vi "RPi HMI Com.vi"(0 "Pump Data":T4={"Voltages"=[0.0, 0.05908203125, 0.06982421875, 0.05908203125, 0.06982421875, 0.0859375], "PumpCurrent"=[0.0015967955457961394, 0.0015950073791676203, 0.0015981739242389562, 0.0015920643549248493, 0.001590499709124895, 0.0015808510600251774], "Speed"=[0.0, 0.0, 0.0, 0.0, 0.0, 0.0], "ControllerCurrent"=[0.0, 0.0, 0.0, 0.0, 0.0, 0.0], "Pressure"=[0.0, 0.0, 0.0, 0.0, 0.0, 0.0], "Flow"=[0.0, 0.0, 0.0, 0.0, 0.0, 0.0], "Elapsed Time:"=[4074.9003000000002, 4074.9003000000002, 4074.9003000000002, 4074.9003000000002, 4074.9003000000002, 4074.9003000000002]} {"Elapsed Time:" format="%<%H:%M:%S>t"; "Speed" format="%#_4f"; "ControllerCurrent" format="%#.1g"; "Pressure" format="%#.0f"; "Flow" format="%#.0f"; "PumpCurrent" format="%#.1g"; "Voltages" format="%#.0f"}, 1 "Tank Data":T10 {"PS Actual (V):" format="%.2f"; "Temp1" format="%#_2g"; "Temp2" format="%#_2g"}, 2 "Power Relays":T9, 3 "Pump CMDs":dbl[](array[numeric]), 4 "HMI Header":T5, 5 "Tank CMDs":T6, 7 "HMI Tog Buttons":T7, 8 "RPi HMI Mode":T11, 9 "In Test":bool, 11 "Controller Config":T1) -> (14 "HMI Cluster":T3 {"Pump Data"."Elapsed Time:" format="%<%H:%M:%S>t"; "Pump Data"."Speed" format="%#_4f"; "Pump Data"."ControllerCurrent" format="%#.1g"; "Pump Data"."Pressure" format="%#.0f"; "Pump Data"."Flow" format="%#.0f"; "Pump Data"."PumpCurrent" format="%#.1g"; "Pump Data"."Voltages" format="%#.0f"})   [LabVIEW 2013]
uses:
  Controls/RPi HMI Mode.ctl
  Controls/Pump Data.ctl
  Controls/HMI Header.ctl
  Controls/Tank CMDs.ctl
  Controls/HMI Tog Buttons.ctl
  Controls/HMI Cluster.ctl
  Controls/HMI Mom Buttons.ctl
  Controls/Controller Config.ctl
  Type Defs/Controller Names.ctl
  <vilib>/Instr/_visa.llb/VISA Configure Serial Port (Instr).vi
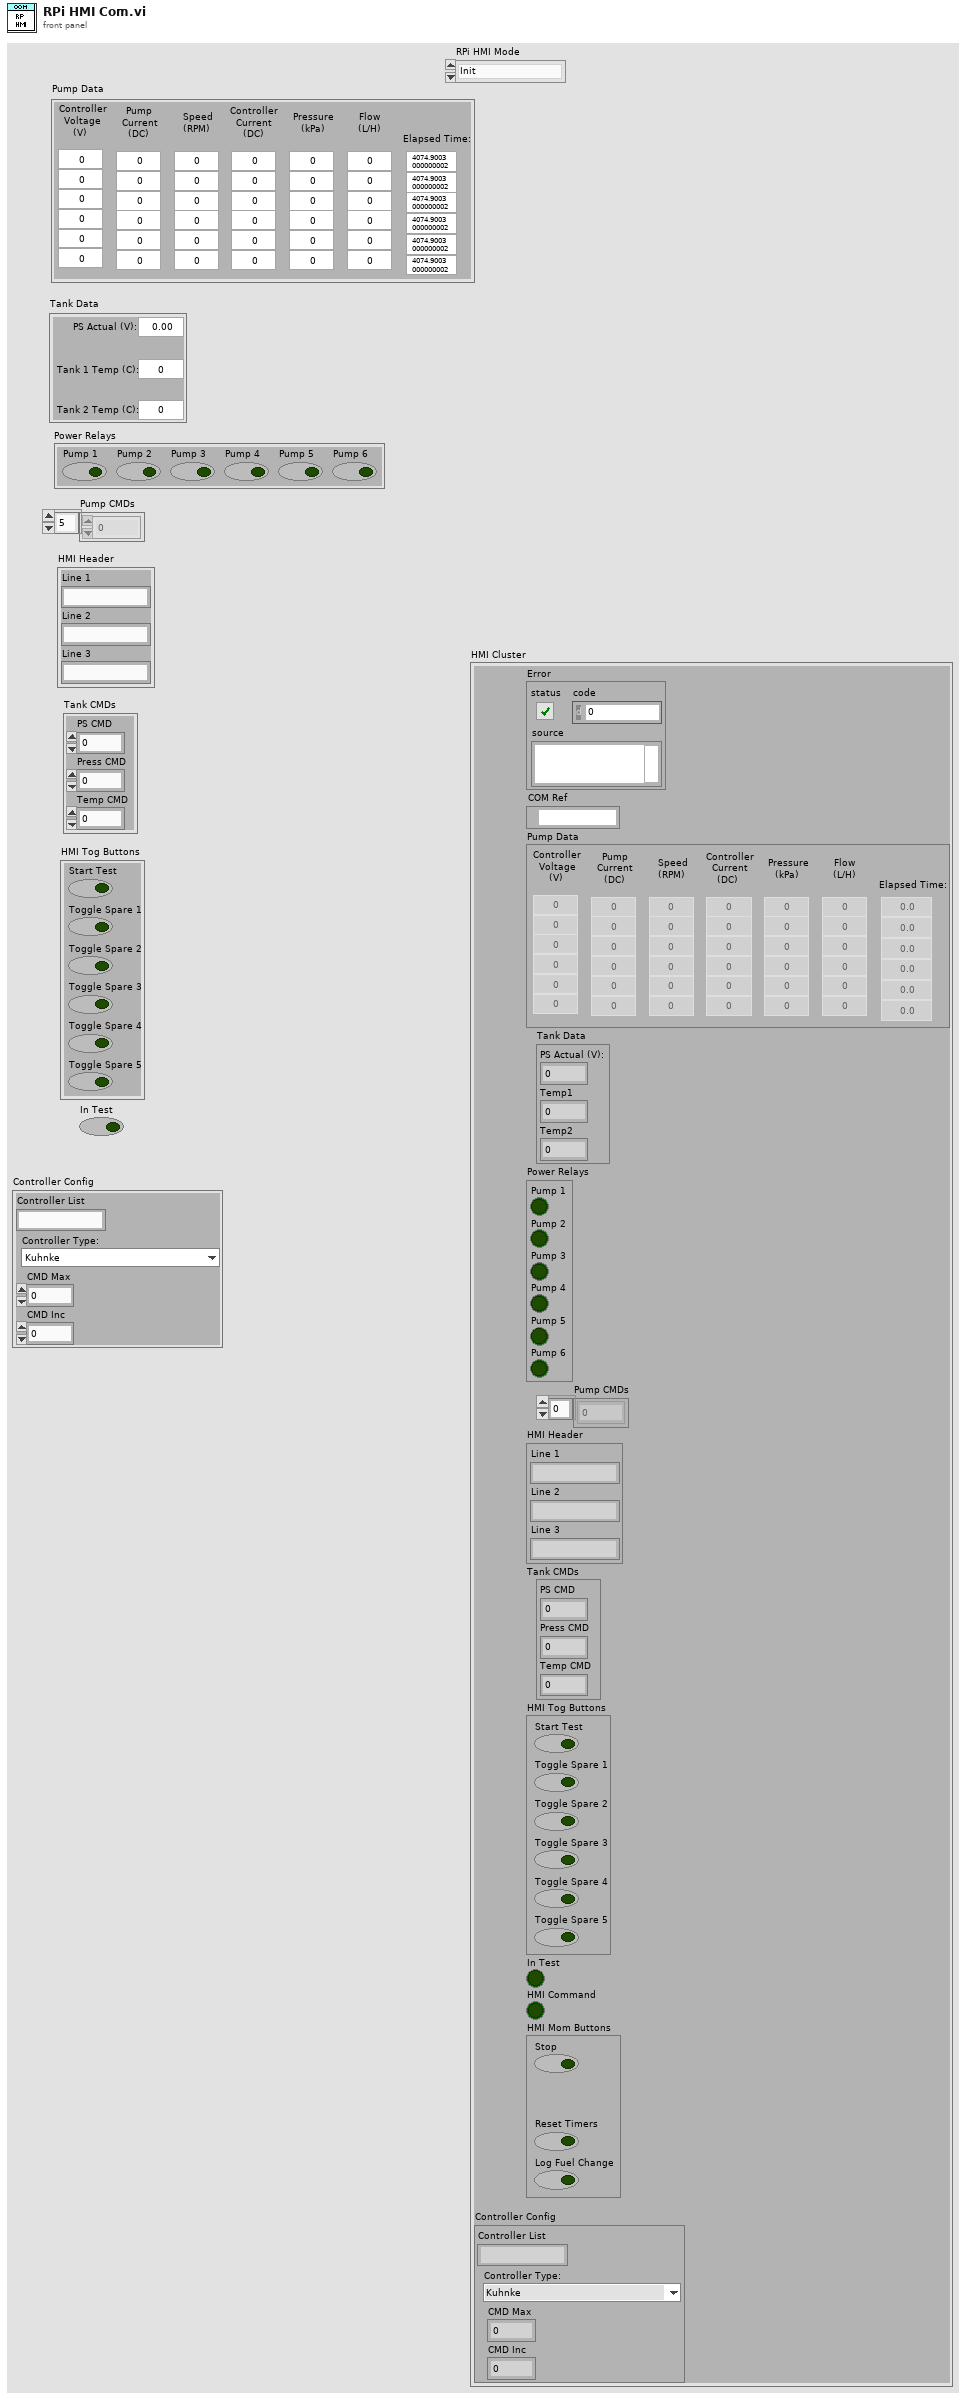
[diagram p1: front panel]
types:
  T1 = typedef "Controller Config.ctl" = cluster{"Controller List":string, "Controller Type:":T2, "CMD Max":i32, "CMD Inc":i32}
  T2 = typedef "Controller Names.ctl" = enum16{"Kuhnke", "Conti", "Hella CAN", "Helbako", "TI PWM", "PSA", "Hella DC Gas", "Hella DC Diesel", "8 Comm", "10 Comm", "8 Comm Hella", "10 Comm Hella", "8 Comm Omron", "10 Comm Omron", "8 Comm Nissan", "10 Comm Nissan"}
  T3 = typedef "HMI Cluster.ctl" = cluster{"Error":errorcluster, "COM Ref":refnum<visa-resource-name>, "Pump Data":T4, "Tank Data":cluster{"PS Actual (V):":dbl, "Temp1":dbl, "Temp2":dbl}, "Power Relays":cluster{"Pump 1":bool, "Pump 2":bool, "Pump 3":bool, "Pump 4":bool, "Pump 5":bool, "Pump 6":bool}, "Pump CMDs":dbl[], "HMI Header":T5, "Tank CMDs":T6, "HMI Tog Buttons":T7, "In Test":bool, "HMI Command":bool, "HMI Mom Buttons":T8, "Controller Config":T1}
  T4 = typedef "Pump Data.ctl" = cluster{"Voltages":dbl[], "PumpCurrent":dbl[], "Speed":dbl[], "ControllerCurrent":dbl[], "Pressure":dbl[], "Flow":dbl[], "Elapsed Time:":dbl[]}
  T5 = typedef "HMI Header.ctl" = cluster{"Line 1":string, "Line 2":string, "Line 3":string}
  T6 = typedef "Tank CMDs.ctl" = cluster{"PS CMD":dbl, "Press CMD":dbl, "Temp CMD":dbl}
  T7 = typedef "HMI Tog Buttons.ctl" = cluster{"Start Test":bool, "Toggle Spare 1":bool, "Toggle Spare 2":bool, "Toggle Spare 3":bool, "Toggle Spare 4":bool, "Toggle Spare 5":bool}
  T8 = typedef "HMI Mom Buttons.ctl" = cluster{"Stop":bool, "Reset Timers":bool, "Log Fuel Change":bool}
  T9 = cluster{"Pump 1":bool, "Pump 2":bool, "Pump 3":bool, "Pump 4":bool, "Pump 5":bool, "Pump 6":bool}
  T10 = cluster{"PS Actual (V):":dbl, "Temp1":dbl, "Temp2":dbl}
  T11 = typedef "RPi HMI Mode.ctl" = enum16{"Init", "Write Data", "Read from RPi", "Write to RPi"}
  T12 = cluster{"Tank CMDs[0]":dbl, "Tank CMDs[1]":dbl, "Tank CMDs[2]":dbl}
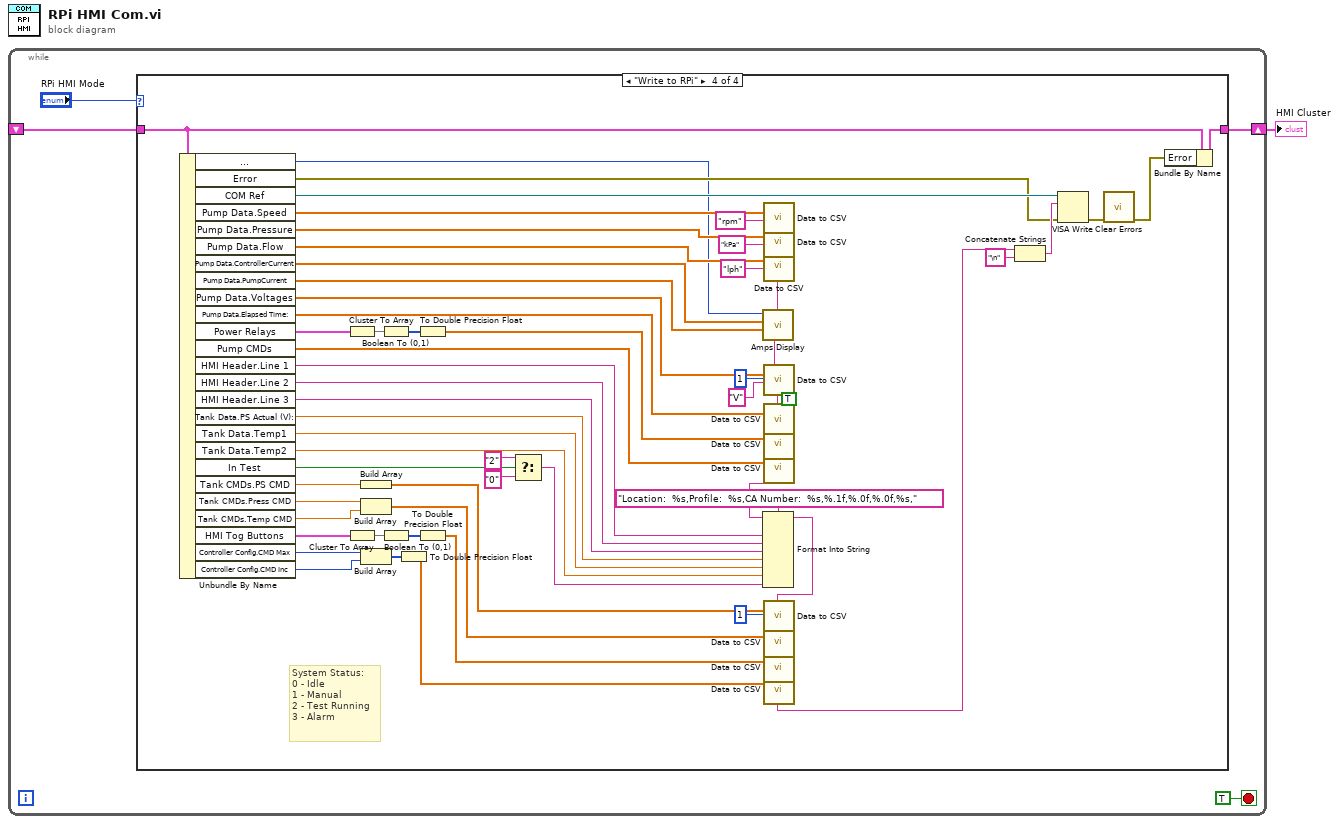
[diagram p0: block diagram]
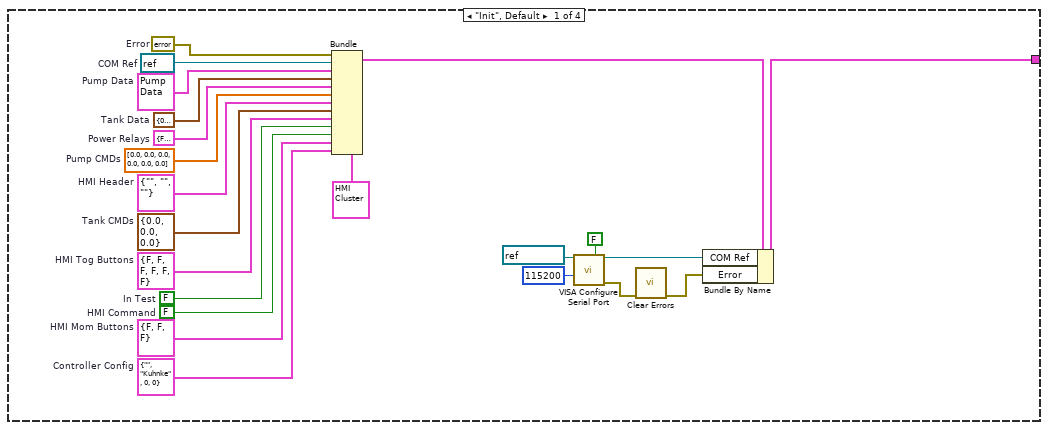
[diagram p2: hidden frame]
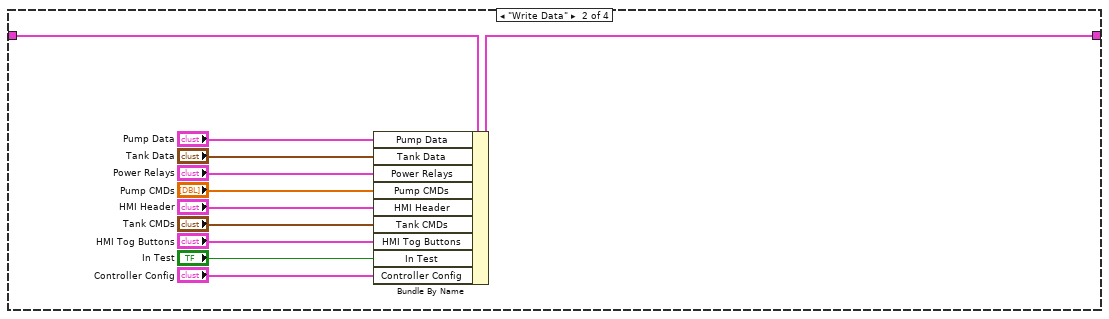
[diagram p3: hidden frame]
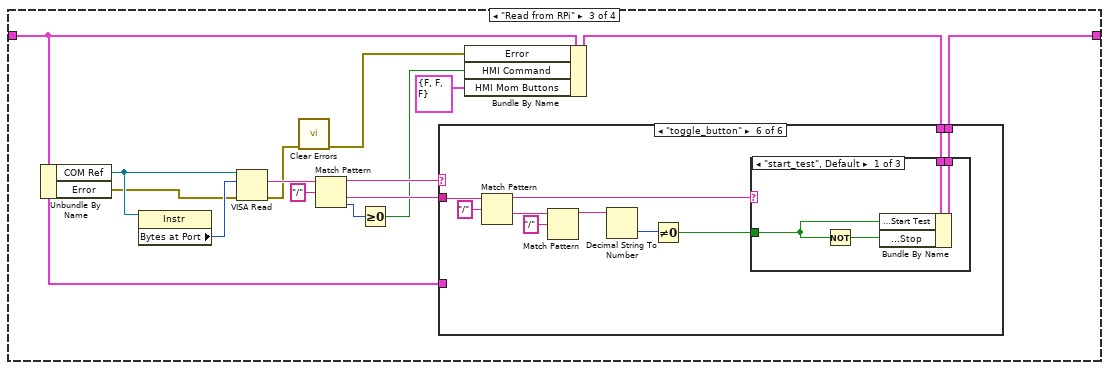
[diagram p4: hidden frame]
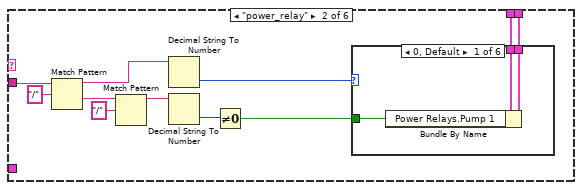
[diagram p6: hidden frame]
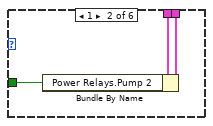
[diagram p7: hidden frame]
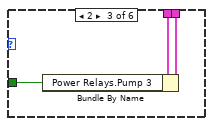
[diagram p8: hidden frame]
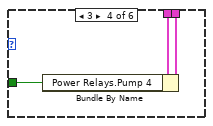
[diagram p9: hidden frame]
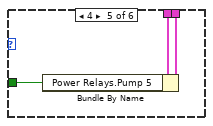
[diagram p10: hidden frame]
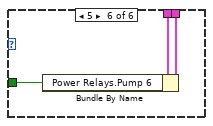
[diagram p11: hidden frame]
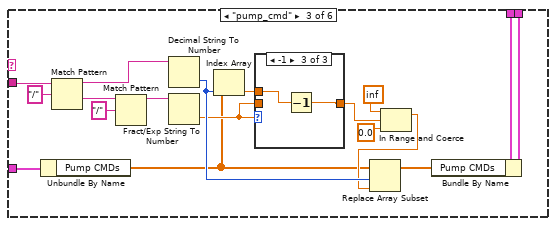
[diagram p12: hidden frame]
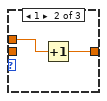
[diagram p14: hidden frame]
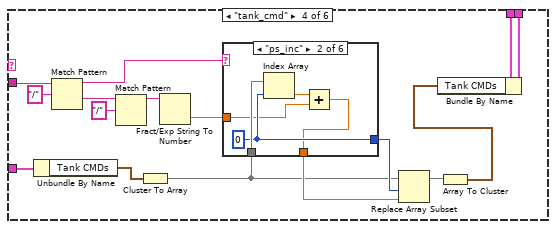
[diagram p15: hidden frame]
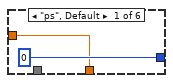
[diagram p16: hidden frame]
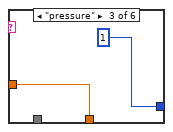
[diagram p17: hidden frame]
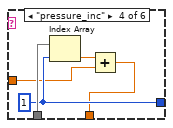
[diagram p18: hidden frame]
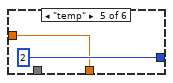
[diagram p19: hidden frame]
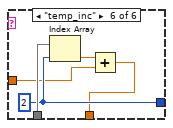
[diagram p20: hidden frame]
diagram:
  n1 = while {
    shift-right: [w3] -> w1
    shift-left: _ -> [w2]
    stop <- TRUE stop-if-true
    n2 = case shown="\"Write to RPi\"" "RPi HMI Mode" {
      tunnel: [w21 w37 w45 w189] -> w3
      tunnel: w2 -> [_ w38 w43 w190]
      frame "Init", Default {
        w6 = T1 {"Controller List"="", "Controller Type:"=enum."Kuhnke", "CMD Max"=0, "CMD Inc"=0}  # Controller Config
        w10 = T8 {"Stop"=FALSE, "Reset Timers"=FALSE, "Log Fuel Change"=FALSE}  # HMI Mom Buttons
        w11 = T9 {"Pump 1"=FALSE, "Pump 2"=FALSE, "Pump 3"=FALSE, "Pump 4"=FALSE, "Pump 5"=FALSE, "Pump 6"=FALSE}  # Power Relays
        w12 = FALSE  # HMI Command
        w13 = FALSE  # In Test
        w14 = T7 {"Start Test"=FALSE, "Toggle Spare 1"=FALSE, "Toggle Spare 2"=FALSE, "Toggle Spare 3"=FALSE, "Toggle Spare 4"=FALSE, "Toggle Spare 5"=FALSE}  # HMI Tog Buttons
        w15 = T6 {"PS CMD"=0.0, "Press CMD"=0.0, "Temp CMD"=0.0}  # Tank CMDs
        w16 = T5 {"Line 1"="", "Line 2"="", "Line 3"=""}  # HMI Header
        w17 = T10 {"PS Actual (V):"=0.0, "Temp1"=0.0, "Temp2"=0.0}  # Tank Data
        w18 = dbl[] [0.0, 0.0, 0.0, 0.0, 0.0, 0.0]  # Pump CMDs
        w19 = errorcluster {"status"=FALSE, "code"=0, "source"=""}  # Error
        w23 = T4 {"Voltages"=[0.0, 0.05908203125, 0.06982421875, 0.05908203125, 0.06982421875, 0.0859375], "PumpCurrent"=[0.0015967955457961394, 0.0015950073791676203, 0.0015981739242389562, 0.0015920643549248493, 0.001590499709124895, 0.0015808510600251774], "Speed"=[0.0, 0.0, 0.0, 0.0, 0.0, 0.0], "ControllerCurrent"=[0.0, 0.0, 0.0, 0.0, 0.0, 0.0], "Pressure"=[0.0, 0.0, 0.0, 0.0, 0.0, 0.0], "Flow"=[0.0, 0.0, 0.0, 0.0, 0.0, 0.0], "Elapsed Time:"=[4074.9003000000002, 4074.9003000000002, 4074.9003000000002, 4074.9003000000002, 4074.9003000000002, 4074.9003000000002]}  # Pump Data
        w24 = refnum<visa-resource-name> refnum  # COM Ref
        n3 = Bundle(cluster=T3 {"Error"={"status"=FALSE, "code"=0, "source"=""}, "COM Ref"="", "Pump Data"={"Voltages"=[], "PumpCurrent"=[], "Speed"=[], "ControllerCurrent"=[], "Pressure"=[], "Flow"=[], "Elapsed Time:"=[]}, "Tank Data"={"PS Actual (V):"=0.0, "Temp1"=0.0, "Temp2"=0.0}, "Power Relays"={"Pump 1"=FALSE, "Pump 2"=FALSE, "Pump 3"=FALSE, "Pump 4"=FALSE, "Pump 5"=FALSE, "Pump 6"=FALSE}, "Pump CMDs"=[], "HMI Header"={"Line 1"="", "Line 2"="", "Line 3"=""}, "Tank CMDs"={"PS CMD"=0.0, "Press CMD"=0.0, "Temp CMD"=0.0}, "HMI Tog Buttons"={"Start Test"=FALSE, "Toggle Spare 1"=FALSE, "Toggle Spare 2"=FALSE, "Toggle Spare 3"=FALSE, "Toggle Spare 4"=FALSE, "Toggle Spare 5"=FALSE}, "In Test"=FALSE, "HMI Command"=FALSE, "HMI Mom Buttons"={"Stop"=FALSE, "Reset Timers"=FALSE, "Log Fuel Change"=FALSE}, "Controller Config"={"Controller List"="", "Controller Type:"=enum."Kuhnke", "CMD Max"=0, "CMD Inc"=0}} ("HMI Cluster"), "Error"=w19, "COM Ref"=w24, "Pump Data"=w23, "Tank Data"=w17, "Power Relays"=w11, "Pump CMDs"=w18, "HMI Header"=w16, "Tank CMDs"=w15, "HMI Tog Buttons"=w14, "In Test"=w13, "HMI Command"=w12, "HMI Mom Buttons"=w10, "Controller Config"=w6) -> (w22:T3)
        n4 = call-poly "VISA Configure Serial Port"("VISA resource name"=refnum<visa-resource-name> "COM1", "Enable Termination\nChar (T)"=FALSE ("Enable Termination\nChar (T)"), "baud rate (9600)"=u32 115200) -> ("VISA resource name out"=w20:refnum<visa-resource-name>, "error out"=w8:errorcluster)  [unwired: 11 in]
        n5 = call <vilib>:"Clear Errors.vi"("error in (no error)"=w8) -> ("error out"=w7:errorcluster)  [unwired: 6 in]
        n6 = Bundle By Name(cluster=w22, "COM Ref"=w20, "Error"=w7) -> (w21:T3)
      }
      frame "Write Data" {
        n7 = Bundle By Name(cluster=w38, "Pump Data"="Pump Data", "Tank Data"="Tank Data", "Power Relays"="Power Relays", "Pump CMDs"="Pump CMDs", "HMI Header"="HMI Header", "Tank CMDs"="Tank CMDs", "HMI Tog Buttons"="HMI Tog Buttons", "In Test"="In Test", "Controller Config"="Controller Config") -> (w37:T3)
      }
      frame "Read from RPi" {
        n8 = Unbundle By Name(w43) -> ("COM Ref"=w50:refnum<visa-resource-name>, "Error"=w41:errorcluster)
        n9 = property class="Instr"(reference=w50) -> ("Bytes at Port"=w51:u32)  [unwired: 1 in, 2 out]
        n10 = VISA Read(VISA resource name=w50, byte count=w51, error in (no error)=w41) -> (read buffer=w52:string, error out=w40:errorcluster)  [unwired: 2 out]
        n11 = call <vilib>:"Clear Errors.vi"("error in (no error)"=w40) -> ("error out"=w39:errorcluster)  [unwired: 6 in]
        n12 = Match Pattern(string=w52, regular expression="/") -> (before substring=w49:string, after substring=w48:string, offset past match=w47:i32)  [unwired: 1 in, 1 out]
        n13 = Greater Or Equal To 0?(x=w47) -> (x >= 0?=w46:bool)
        n14 = Bundle By Name(cluster=w43, "Error"=w39, "HMI Command"=w46, "HMI Mom Buttons"=T8 {"Stop"=FALSE, "Reset Timers"=FALSE, "Log Fuel Change"=FALSE}) -> (w44:T3)
        n15 = case shown="\"toggle_button\"" w49 {
          tunnel: w48 -> [_ w64 w100 w121 w147 w166]
          tunnel: w44 -> [w54 w58 w87 w109 w145 w164]
          tunnel: [w54 w57 w86 w108 w144 w163] -> w45
          tunnel: w43 -> [_ _ w84 w113 _ _]
          frame "null", Default {
          }
          frame "power_relay" {
            n16 = Match Pattern(string=w64, regular expression="/") -> (before substring=w59:string, after substring=w62:string)  [unwired: 1 in, 2 out]
            n17 = Match Pattern(string=w62, regular expression="/") -> (before substring=w61:string)  [unwired: 1 in, 3 out]
            n18 = Decimal String To Number(string=w59) -> (number=w56:i32)  [unwired: 2 in, 1 out]
            n19 = Decimal String To Number(string=w61) -> (number=w60:i32)  [unwired: 2 in, 1 out]
            n20 = Not Equal To 0?(x=w60) -> (x != 0?=w55:bool)
            n21 = case shown="0, Default" w56 {
              tunnel: w58 -> [w68 w71 w74 w77 w80 w83]
              tunnel: [w67 w70 w73 w76 w79 w82] -> w57
              tunnel: w55 -> [w66 w69 w72 w75 w78 w81]
              frame 0, Default {
                n22 = Bundle By Name(cluster=w68, "Power Relays.Pump 1"=w66) -> (w67:T3)
              }
              frame 1 {
                n23 = Bundle By Name(cluster=w71, "Power Relays.Pump 2"=w69) -> (w70:T3)
              }
              frame 2 {
                n24 = Bundle By Name(cluster=w74, "Power Relays.Pump 3"=w72) -> (w73:T3)
              }
              frame 3 {
                n25 = Bundle By Name(cluster=w77, "Power Relays.Pump 4"=w75) -> (w76:T3)
              }
              frame 4 {
                n26 = Bundle By Name(cluster=w80, "Power Relays.Pump 5"=w78) -> (w79:T3)
              }
              frame 5 {
                n27 = Bundle By Name(cluster=w83, "Power Relays.Pump 6"=w81) -> (w82:T3)
              }
            }
          }
          frame "pump_cmd" {
            n28 = Unbundle By Name(w84) -> ("Pump CMDs"=w88:dbl[])
            n29 = Match Pattern(string=w100, regular expression="/") -> (before substring=w96:string, after substring=w98:string)  [unwired: 1 in, 2 out]
            n30 = Match Pattern(string=w98, regular expression="/") -> (before substring=w97:string)  [unwired: 1 in, 3 out]
            n31 = Decimal String To Number(string=w96) -> (number=w94:i32)  [unwired: 2 in, 1 out]
            n32 = Fract/Exp String To Number(string=w97) -> (number=w93:dbl)  [unwired: 3 in, 1 out]
            n33 = Index Array(array=w88, index=w94) -> (element=w95:dbl)
            n34 = case shown="-1" w93 {
              tunnel: w95 -> [_ w104 w106]
              tunnel: w93 -> [w102 _ _]
              tunnel: [w102 w103 w105] -> w92
              frame 0, Default {
              }
              frame 1 {
                n35 = Increment(x=w104) -> (x+1=w103:dbl)
              }
              frame -1 {
                n36 = Decrement(x=w106) -> (x-1=w105:dbl)
              }
            }
            n37 = In Range and Coerce(upper limit=inf, x=w92, lower limit=0.0) -> (coerced(x)=w89:dbl)  [unwired: 1 out]
            n38 = Replace Array Subset(array=w88, new element=w89, index=w94) -> (w85:dbl[])
            n39 = Bundle By Name(cluster=w87, "Pump CMDs"=w85) -> (w86:T3)
          }
          frame "tank_cmd" {
            n40 = Unbundle By Name(w113) -> ("Tank CMDs"=w112:T6)
            n41 = Match Pattern(string=w121, regular expression="/") -> (before substring=w117:string, after substring=w119:string)  [unwired: 1 in, 2 out]
            n42 = Match Pattern(string=w119, regular expression="/") -> (before substring=w118:string)  [unwired: 1 in, 3 out]
            n43 = Cluster To Array(cluster=w112) -> (array=w111:dbl[])
            n44 = Fract/Exp String To Number(string=w118) -> (number=w114:dbl)  [unwired: 3 in, 1 out]
            n45 = case shown="\"ps_inc\"" w117 {
              tunnel: [0 w128 1 w135 2 w142] -> w116
              tunnel: [w123 w125 w130 w132 w137 w139] -> w115
              tunnel: w114 -> [w123 w126 w130 w133 w137 w140]
              tunnel: w111 -> [_ w129 _ w136 _ w143]
              frame "ps", Default {
              }
              frame "ps_inc" {
                w128 = 0
                n46 = Index Array(array=w129, index=w128) -> (element=w127:dbl)
                n47 = Add(x=w127, y=w126) -> (x+y=w125:dbl)
              }
              frame "pressure" {
              }
              frame "pressure_inc" {
                w135 = 1
                n48 = Index Array(array=w136, index=w135) -> (element=w134:dbl)
                n49 = Add(x=w134, y=w133) -> (x+y=w132:dbl)
              }
              frame "temp" {
              }
              frame "temp_inc" {
                w142 = 2
                n50 = Index Array(array=w143, index=w142) -> (element=w141:dbl)
                n51 = Add(x=w141, y=w140) -> (x+y=w139:dbl)
              }
            }
            n52 = Replace Array Subset(array=w111, new element=w115, index=w116) -> (w110:dbl[])
            n53 = Array To Cluster(array=w110) -> (cluster=w107:T12)
            n54 = Bundle By Name(cluster=w109, "Tank CMDs"=w107) -> (w108:T3)
          }
          frame "momentary_button" {
            n55 = Match Pattern(string=w147, regular expression="/") -> (before substring=w146:string)  [unwired: 1 in, 3 out]
            n56 = case shown="\"reset_timers\"" w146 {
              tunnel: w145 -> [w151 w153 w156]
              tunnel: [w150 w152 w155] -> w144
              frame "stop", Default {
                n57 = Bundle By Name(cluster=w151, "HMI Mom Buttons.Stop"=TRUE) -> (w150:T3)
              }
              frame "reset_timers" {
                n58 = Bundle By Name(cluster=w153, "HMI Mom Buttons.Reset Timers"=TRUE ("HMI Mom Buttons.Stop")) -> (w152:T3)
              }
              frame "log_fuel_change" {
                n59 = Bundle By Name(cluster=w156, "HMI Mom Buttons.Log Fuel Change"=TRUE ("HMI Mom Buttons.Stop")) -> (w155:T3)
              }
            }
          }
          frame "toggle_button" {
            n60 = Match Pattern(string=w166, regular expression="/") -> (before substring=w165:string, after substring=w161:string)  [unwired: 1 in, 2 out]
            n61 = Match Pattern(string=w161, regular expression="/") -> (before substring=w159:string)  [unwired: 1 in, 3 out]
            n62 = Decimal String To Number(string=w159) -> (number=w160:i32)  [unwired: 2 in, 1 out]
            n63 = Not Equal To 0?(x=w160) -> (x != 0?=w158:bool)
            n64 = case shown="\"start_test\", Default" w165 {
              tunnel: w164 -> [w171 w173 w176]
              tunnel: [w170 w172 w175] -> w163
              tunnel: w158 -> [w169 _ _]
              frame "start_test", Default {
                n65 = Not(x=w169) -> (.not. x?=w168:bool)
                n66 = Bundle By Name(cluster=w171, "HMI Tog Buttons.Start Test"=w169, "HMI Mom Buttons.Stop"=w168) -> (w170:T3)
              }
              frame "reset_timers" {
                n67 = Bundle By Name(cluster=w173, "HMI Mom Buttons.Reset Timers"=TRUE ("HMI Mom Buttons.Stop")) -> (w172:T3)
              }
              frame "log_fuel_change" {
                n68 = Bundle By Name(cluster=w176, "HMI Mom Buttons.Log Fuel Change"=TRUE ("HMI Mom Buttons.Stop")) -> (w175:T3)
              }
            }
          }
        }
      }
      frame "Write to RPi" {
        # "System Status:\n0 - Idle\n1 - Manual\n2 - Test Running\n3 - Alarm"
        n69 = Unbundle By Name(w190) -> ("Controller Config.Controller Type:"=w178:T2, "Error"=w191:errorcluster, "COM Ref"=w240:refnum<visa-resource-name>, "Pump Data.Speed"=w239:dbl[], "Pump Data.Pressure"=w231:dbl[], "Pump Data.Flow"=w230:dbl[], "Pump Data.ControllerCurrent"=w229:dbl[], "Pump Data.PumpCurrent"=w228:dbl[], "Pump Data.Voltages"=w227:dbl[], "Pump Data.Elapsed Time:"=w224:dbl[], "Power Relays"=w193:T9, "Pump CMDs"=w222:dbl[], "HMI Header.Line 1"=w218:string, "HMI Header.Line 2"=w217:string, "HMI Header.Line 3"=w216:string, "Tank Data.PS Actual (V):"=w215:dbl, "Tank Data.Temp1"=w214:dbl, "Tank Data.Temp2"=w213:dbl, "In Test"=w212:bool, "Tank CMDs.PS CMD"=w206:dbl, "Tank CMDs.Press CMD"=w205:dbl, "Tank CMDs.Temp CMD"=w204:dbl, "HMI Tog Buttons"=w200:T7, "Controller Config.CMD Max"=w186:i32, "Controller Config.CMD Inc"=w185:i32)
        n70 = Cluster To Array(cluster=w193) -> (array=w194:bool[])
        n71 = Cluster To Array(cluster=w200) -> (array=w199:bool[])
        n72 = Build Array(w206) -> (w203:dbl[])
        n73 = Build Array(w205, w204) -> (w201:dbl[])
        n74 = Build Array(w186, w185) -> (w184:i32[])
        n75 = Boolean To (0,1)(Boolean=w194) -> (0, 1=w195:i16[])
        n76 = Boolean To (0,1)(Boolean=w199) -> (0, 1=w198:i16[])
        n77 = To Double Precision Float(number=w184) -> (double precision float=w182:dbl[])
        n78 = To Double Precision Float(number=w195) -> (double precision float=w192:dbl[])
        n79 = To Double Precision Float(number=w198) -> (double precision float=w197:dbl[])
        n80 = Select(t="2" ("Units"), s=w212, f="0" ("Units")) -> (s? t:f=w209:string)
        n81 = call "Data to CSV.vi"("Data Array"=w239, "Units"="rpm") -> ("String OUT"=w233:string)  [unwired: 25 in]
        n82 = call "Data to CSV.vi"("Data Array"=w231, "Units"="kPa", "String IN"=w233) -> ("String OUT"=w232:string)  [unwired: 24 in]
        n83 = call "Data to CSV.vi"("Data Array"=w230, "Units"="lph", "String IN"=w232) -> ("String OUT"=w180:string)  [unwired: 24 in]
        n84 = call "Amps Display.vi"("String IN"=w180, "Pump Current"=w228, "Controller Current"=w229, "Controller Type:"=w178) -> ("String OUT"=w179:string)  [unwired: 7 in]
        n85 = call "Data to CSV.vi"("Data Array"=w227, "Precision (0)"=i16 1, "Units"="V", "String IN"=w179) -> ("String OUT"=w225:string)  [unwired: 23 in]
        n86 = call "Data to CSV.vi"("Data Array"=w224, "String IN"=w225, "Time? (F)"=TRUE) -> ("String OUT"=w223:string)  [unwired: 24 in]
        n87 = call "Data to CSV.vi"("Data Array"=w192, "String IN"=w223) -> ("String OUT"=w221:string)  [unwired: 25 in]
        n88 = call "Data to CSV.vi"("Data Array"=w222, "String IN"=w221) -> ("String OUT"=w220:string)  [unwired: 25 in]
        n89 = Format Into String(format string="Location:  %s,Profile:  %s,CA Number:  %s,%.1f,%.0f,%.0f,%s,", initial string=w220, w218, w217, w216, w215, w214, w213, w209) -> (resulting string=w207:string)  [unwired: 1 in, 1 out]
        n90 = call "Data to CSV.vi"("Data Array"=w203, "Precision (0)"=i16 1, "String IN"=w207) -> ("String OUT"=w202:string)  [unwired: 24 in]
        n91 = call "Data to CSV.vi"("Data Array"=w201, "String IN"=w202) -> ("String OUT"=w196:string)  [unwired: 25 in]
        n92 = call "Data to CSV.vi"("Data Array"=w197, "String IN"=w196) -> ("String OUT"=w183:string)  [unwired: 25 in]
        n93 = call "Data to CSV.vi"("Data Array"=w182, "String IN"=w183) -> ("String OUT"=w181:string)  [unwired: 25 in]
        n94 = Concatenate Strings(w181, "\n" ("string")) -> (w242:string)
        n95 = VISA Write(VISA resource name=w240, write buffer=w242, error in (no error)=w191) -> (error out=w188:errorcluster)  [unwired: 2 out]
        n96 = call <vilib>:"Clear Errors.vi"("error in (no error)"=w188) -> ("error out"=w187:errorcluster)  [unwired: 6 in]
        n97 = Bundle By Name(cluster=w190, "Error"=w187) -> (w189:T3)
      }
    }
  }
  "HMI Cluster" <- w1
